vi "Remote Shutdown Status.vi"() -> (2 "Subsystem Status":T1)   [LabVIEW 2015]
uses:
  Vehicle Status/Subsystem Status.ctl
  Vehicle Status/Subsystem Status Severity.ctl
  Vehicle Status/Subsystem Status Message.ctl
  Global Data.vi
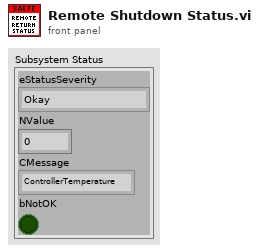
[diagram p1: front panel]
types:
  T1 = typedef "Subsystem Status.ctl" = cluster{"eStatusSeverity":T2, "NValue":sgl, "CMessage":T3, "bNotOK":bool}
  T2 = typedef "Subsystem Status Severity.ctl" = enum16{"Okay", "Short Warning", "Long Warning", "Return to Pits", "Error", "Danger"}
  T3 = typedef "Subsystem Status Message.ctl" = enum16{"ControllerTemperature", "MotorTemperature", "BatteryTemperature", "BatteryLowVoltage", "LVBattery", "sbRIOTemperature", "Precharge", "BSPD", "IMD", "RemoteReturnToPits", "EStopInterrupted", "NoCellComms", "MCOverSpeed", "MCOverCurrent", "MCOverVoltage", "MCInverterOverTemp", "MCDirectionCommand", "MCInverterTimeout", "MCDesatFault", "MCHWOverCurrent", "MCUnderVoltage", "MCCommandMessageLost", "MotorOverTemp", "MCModAOverTemp", "MCModBOverTemp", "MCModCOverTemp", "MCPCBOverTemp", "MCGateDrv1OverTemp", "MCDateDrv2OverTemp", "MCCurrentSensorFault", "MCResolverNotConnected", "ShutdownLatchTripped", "UnknownBMS", "RemoteEmergency"}
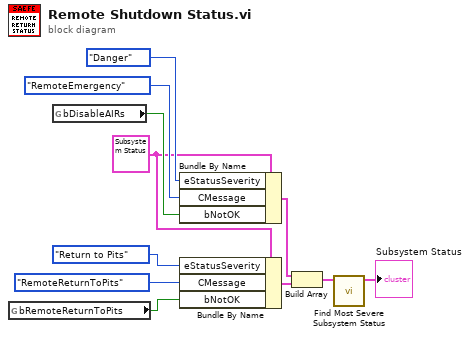
[diagram p0: block diagram]
diagram:
  w7 = T1 {"eStatusSeverity"=enum."Okay", "NValue"=0.0, "CMessage"=enum."ControllerTemperature", "bNotOK"=FALSE} ("Subystem Status")
  n1 = global read "Global Data.vi" "bRemoteReturnToPits"() -> (w6:bool)
  n2 = global read "Global Data.vi" "bDisableAIRs"() -> (w10:bool)
  n3 = Bundle By Name(cluster=w7, "eStatusSeverity"=Subsystem_Status_Severity."Danger" ("Status Severity"), "CMessage"=Subsystem_Status_Message."RemoteEmergency" ("Message"), "bNotOK"=w10) -> (w3:T1)
  n4 = Bundle By Name(cluster=w7, "eStatusSeverity"=Subsystem_Status_Severity."Return to Pits" ("Status Severity"), "CMessage"=Subsystem_Status_Message."RemoteReturnToPits" ("Message"), "bNotOK"=w6) -> (w2:T1)
  n5 = Build Array(w3, w2) -> (w1:T1[])
  n6 = call "Find Most Severe Subsystem Status.vi"("Array"=w1) -> ("Subystem Status"=→"Subsystem Status":T1)  [unwired: 10 in]
